vi "Composed Context to Default.vi"(8 "error in":errorcluster, 11 "State in":refnum<class "State Pattern.lvclass">) -> (0 "error out":errorcluster, 3 "State out":refnum<class "State Pattern.lvclass">)   [LabVIEW 2021, in "State Pattern.lvclass"]
uses:
  State Pattern.lvclass
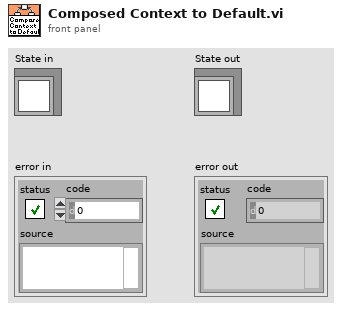
[diagram p1: front panel]
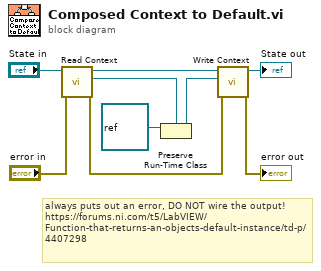
[diagram p0: block diagram]
diagram:
  # "always puts out an error, DO NOT wire the output!\nhttps://forums.ni.com/t5/LabVIEW/Function-that-returns-an-objects-default-instance/td-p/4407298"
  n1 = call-dynamic "Read Context.vi"("error in"="error in", "State in"="State in") -> ("error out"=w8:errorcluster, "Context"=w2:refnum<class "State Pattern.lvclass">, "State out"=w9:refnum<class "State Pattern.lvclass">)  [unwired: 7 in]
  n2 = Preserve Run-Time Class(object in=refnum<class> refnum ("LabVIEW Object"), 2:w2) -> (object out=w1:refnum<class "State Pattern.lvclass">)  [unwired: 1 in, 1 out]
  n3 = call-dynamic "Write Context.vi"("error in"=w8, "Context"=w1, "State in"=w9) -> ("error out"=→"error out":errorcluster, "State out"=→"State out":refnum<class "State Pattern.lvclass">)  [unwired: 7 in]
